vi "AddDependency.vi"(8 "error in (no error)":errorcluster, 9 "Item to depend on":refnum<class "ILabVIEWItem.lvclass">, 11 "CLabVIEWItem in":refnum<class "CLabVIEWItem.lvclass">) -> (0 "error out":errorcluster, 3 "CLabVIEWItem out":refnum<class "CLabVIEWItem.lvclass">)   [LabVIEW 2020, in "LabVIEWItem.lvlib" / "CLabVIEWItem.lvclass"]
uses:
  CLabVIEWItem.lvclass
  obj/Addons/LabVIEWObjectInterfaces.lvlibp/LabVIEWObjectInterfaces/ILabVIEWItem/ILabVIEWItem.lvclass
  CLabVIEWItem.lvclass/CLabVIEWItem.ctl
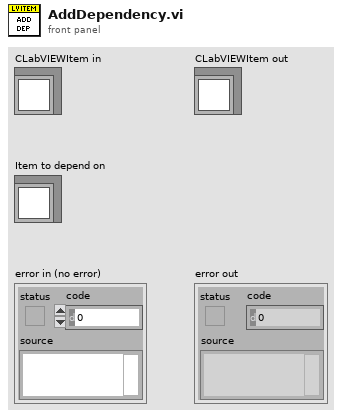
[diagram p1: front panel]
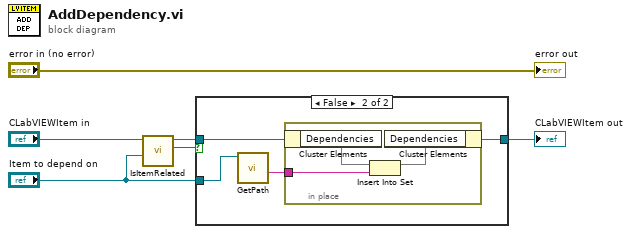
[diagram p0: block diagram]
diagram:
  n1 = call-dynamic "IsItemRelated.vi"("Item to compare"="Item to depend on", "CLabVIEWItem in"="CLabVIEWItem in") -> ("Is item related?"=w1:bool, "CLabVIEWItem out"=w3:refnum<class "CLabVIEWItem.lvclass">)  [unwired: 7 in, 1 out]
  n2 = case shown="False" w1 {
    tunnel: [w7 w11] -> w6
    tunnel: w3 -> [w7 w10]
    tunnel: "Item to depend on" -> [_ w8]
    frame True {
    }
    frame False {
      n3 = call-dynamic "GetPath.vi"("ILabVIEWItem in"=w8) -> ("Path"=w9:string)  [unwired: 8 in, 2 out]
      n4 = in-place {
        in-place-border: w9 -> [w12]
        n5 = in-place-cluster #1(w10) -> ("Dependencies"=w14:set{string})
        n6 = Insert Into Set(10:w12, 11:w14) -> (3:w13:set{string})  [unwired: 1 out]
        n7 = in-place-cluster #1("Dependencies"=w13) -> (w11:refnum<class "CLabVIEWItem.lvclass">)
      }
    }
  }
  "CLabVIEWItem out" <- w6
  "error out" <- "error in (no error)"
